vi "gen_array.vi"(0 "rows":dbl, 2 "columns":dbl) -> (1 "Array":dbl[][](array[numeric]) format="%#_4g")   [LabVIEW 2023]
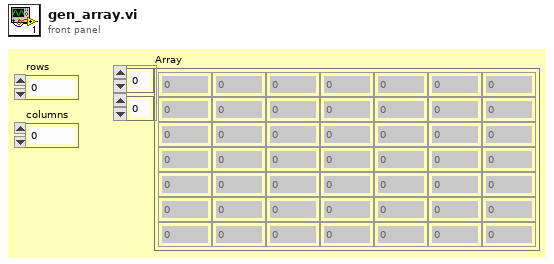
[diagram p1: front panel]
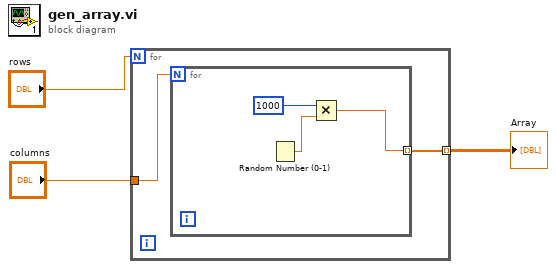
[diagram p0: block diagram]
diagram:
  n1 = for {
    N: "rows" -> [_]
    tunnel: [w5] -> w2 mode=indexing
    tunnel: "columns" -> [w4]
    n2 = for {
      N: w4 -> [_]
      tunnel: [w6] -> w5 mode=indexing
      n3 = Random Number (0-1)() -> (number: 0 to 1=w7:dbl)
      n4 = Multiply(x=1000, y=w7) -> (x*y=w6:dbl)
    }
  }
  "Array" <- w2
